vi "NI Vision Camera.vi"   [LabVIEW 2014]
uses:
  Project/Implementations/Hardware/Real Hardware/ReadoutDevice/NI Vision Camera/NI Vision Camera.lvclass
  <vilib>/ActorFramework/Actor/Actor.lvclass
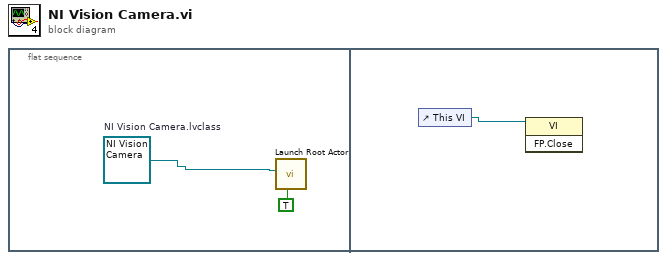
[diagram p0: block diagram]
diagram:
  n1 = flat-sequence {
    frame #0 {
      w1 = refnum<class "NI Vision Camera.lvclass"> refnum  # NI Vision Camera.lvclass
      n2 = call <vilib>:"Launch Root Actor.vi"("Open Actor Core front panel? (F)"=TRUE, "Actor"=w1) -> ()  [unwired: 8 in, 2 out]
    }
    frame #1 {
      n3 = control-ref of="This VI"() -> (w3:refnum<vi>)
      n4 = invoke class="VI" method="FP.Close"(reference=w3) -> ()  [unwired: 2 in, 3 out]
    }
  }
